vi "panel.vi"() -> ()   [LabVIEW 2018]
panel:
  out "?":string
  out "?":string
  out "?":string
  out "Komunikaty":string
  out "ERROR":bool
  in  "ON/OFF":bool
  out "mbar":dbl
  out "ON":bool
  out "Ciśnienie":dbl(slide) scale=0.0..1013.0
  in  "stop":bool
  in  "ON/OFF":bool
  out "Skład procentowy gazów":waveform(dbl)(graph)
  out "Ciśninie w komorze":waveform(dbl)(graph)
  out "Obciążenie":dbl(knob) scale=0.0..100.0
  out "ON":bool
  in  "?":T1(tab)
  in  "?":bool
  in  "Gaz 3":string(combo)
  out "Urządzenie:":string
  in  "Włącz":bool
  out "Sprawny":bool
  in  "Przepływ":dbl(slide) scale=0.0..10.0
  in  "?":bool
  in  "Gaz":string(combo)
  out "Urządzenie:":string
  in  "Włącz":bool
  out "Sprawny 2":bool
  in  "Przepływ":dbl(slide) scale=0.0..10.0
  in  "Przepływ":dbl(slide) scale=0.0..10.0
  out "Sprawny":bool
  in  "Włącz":bool
  out "Urządzenie:":string
  in  "Gaz":string(combo)
  in  "?":bool
  out "ON":bool
  out "ON":bool
  out "ON":bool
  out "Ring":u16(ring)
  out "?":dbl(slide) scale=0.0..100.0
  out "?":dbl(slide) scale=0.0..100.0
  out "?":dbl(slide) scale=0.0..100.0
  # "MIESZALNIK GAZOWY"
  # "MANOMETR"
  # "POMPA PRӯNIOWA"
  # "KOMORA EKSPERYMENTALNA"
  # "PROGRAM"
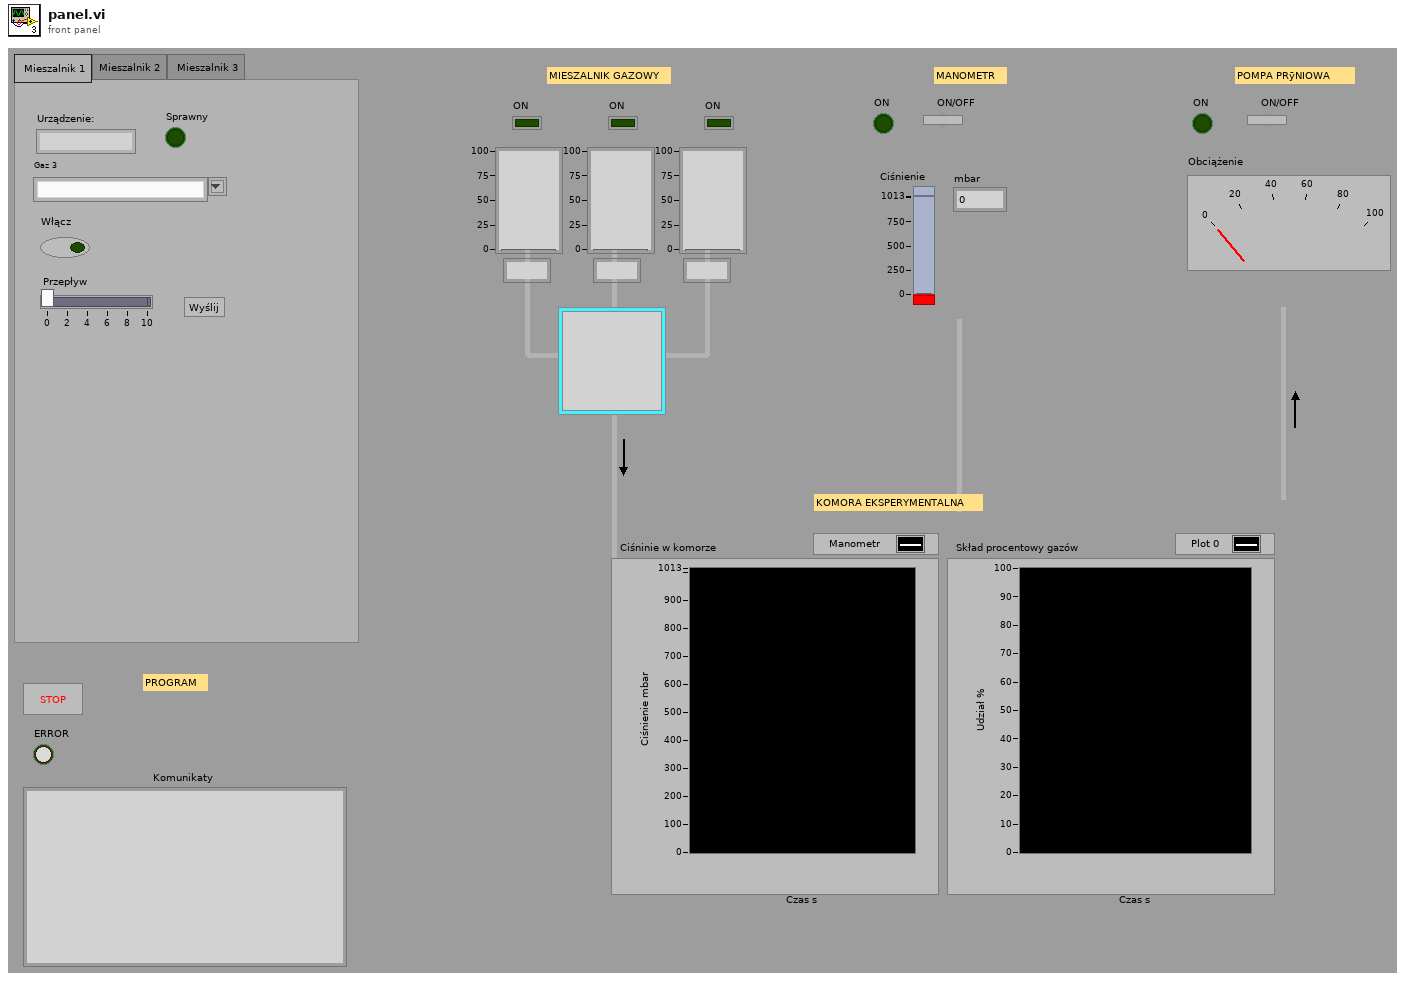
[diagram p1: front panel]
types:
  T1 = enum32{" Mieszalnik 1", "Mieszalnik 2", " Mieszalnik 3"}
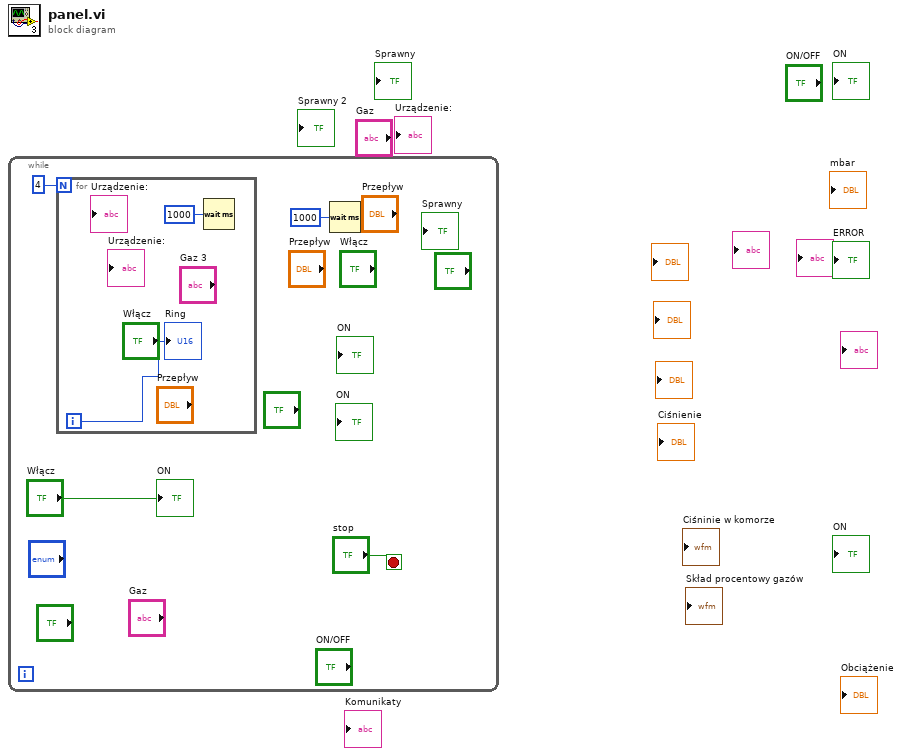
[diagram p0: block diagram]
diagram:
  n1 = while {
    stop <- "stop" stop-if-true
    n2 = for {
      N: 4 -> [_]
      i -> [w5]
      n3 = Wait (ms)(milliseconds to wait=u32 1000) -> ()  [unwired: 1 out]
      "Ring" <- w5
    }
    n4 = Wait (ms)(milliseconds to wait=u32 1000) -> ()  [unwired: 1 out]
    "ON" <- "Włącz"
  }
